vi "Update Clock Map.vi"(7 "Reset":bool, 9 "ClockID":u8, 10 "Timestamp Pair":T1, 11 "Clock History Map in":T3) -> (3 "Clock History Map out":map{u8, T2}(c390))   [LabVIEW 2021, in "CIFClocks.lvlib"]
uses:
  CIFClocks.lvlib
  Typedef/Clock History Map.ctl
  Typedef/Clock History.ctl
  Typedef/Timestamp Pair.ctl
  <vilib>/Utility/miscctls.llb/LVMapReplaceAction.ctl
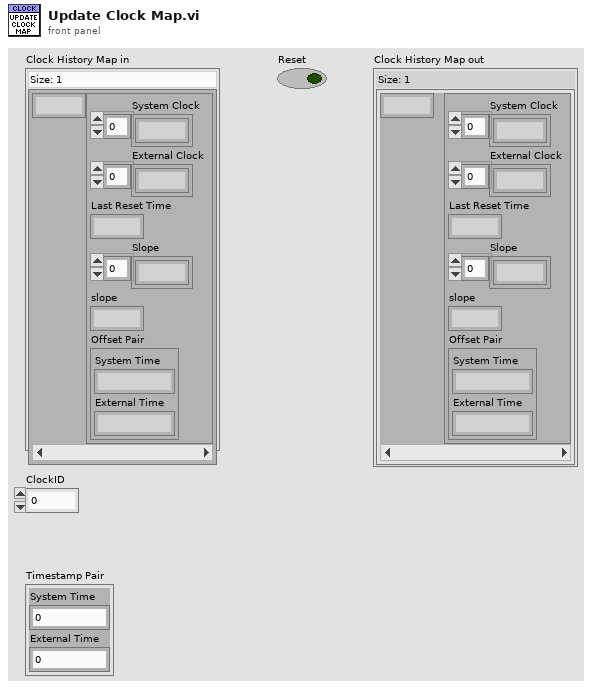
[diagram p1: front panel]
types:
  T1 = typedef "CIFClocks.lvlib/Timestamp Pair.ctl" = cluster{"System Time":i64, "External Time":i64}
  T2 = typedef "CIFClocks.lvlib/Clock History.ctl" = cluster{"System Clock":i64[], "External Clock":i64[], "Last Reset Time":u64, "Slope":dbl[], "slope":dbl, "Offset Pair":T1}
  T3 = typedef "CIFClocks.lvlib/Clock History Map.ctl" = map{u8, T2}
  T4 = typedef "LVMapReplaceAction.ctl" = enum32{"Modify Entry only if found", "Add or Modify Entry", "Delete Entry"}
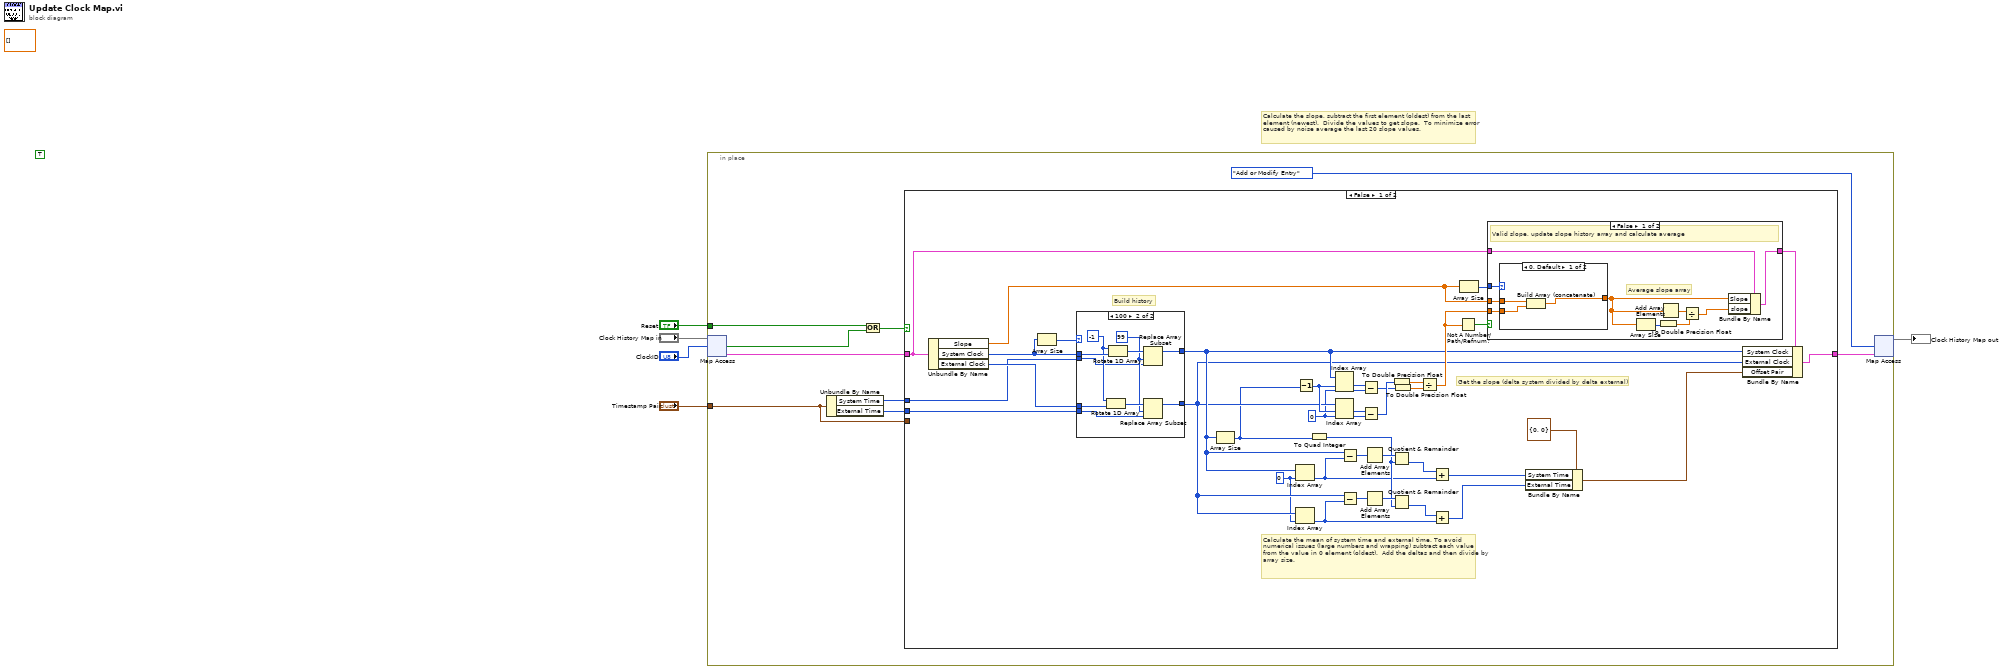
[diagram p0: block diagram]
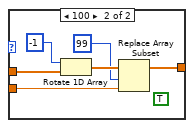
[diagram p2: hidden frame]
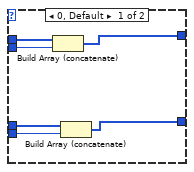
[diagram p4: hidden frame]
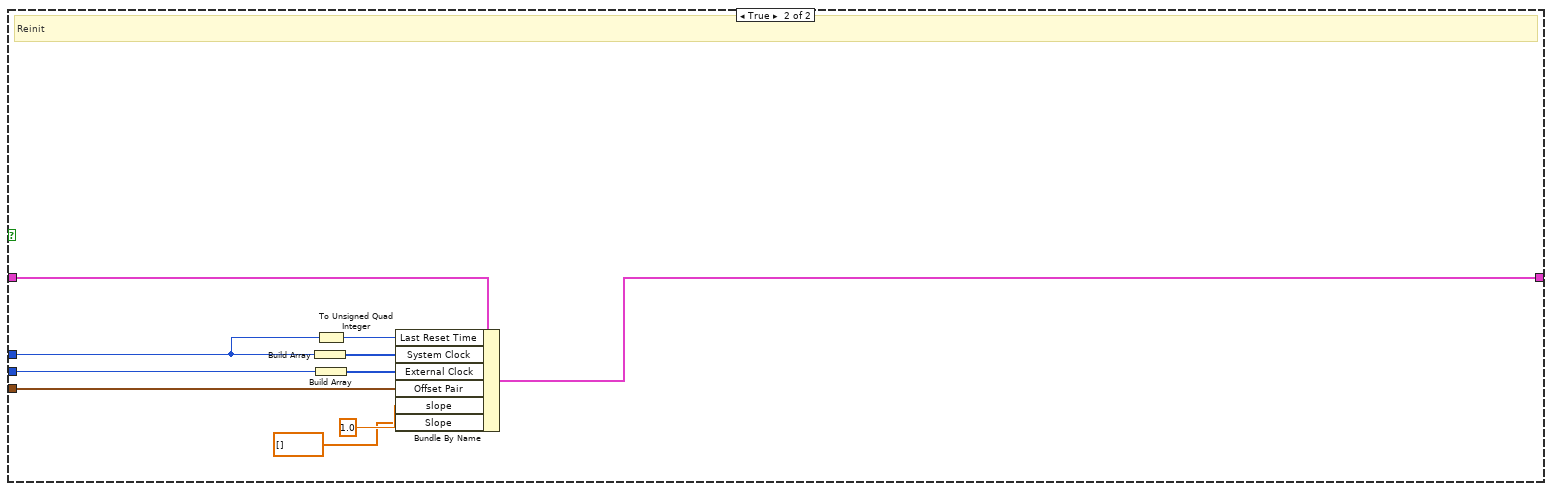
[diagram p5: hidden frame]
diagram:
  (unwired) TRUE
  (unwired) dbl[][] []
  # "Calculate the slope, subtract the first element (oldest) from the last element (newest).  Divide the values to get slope.  To minimize error caused by noise average the last 20 slope values."
  n1 = in-place {
    in-place-border: "Timestamp Pair" -> [w6]
    in-place-border: "Reset" -> [w13]
    n2 = in-place-map #1("Clock History Map in", "ClockID") -> (w11:T2, w14:bool)  [unwired: 1 in]
    n3 = Unbundle By Name(w6) -> ("System Time"=w8:i64, "External Time"=w7:i64)
    n4 = Or(x=w13, y=w14) -> (x .or. y?=w12:bool)
    n5 = case shown="False" w12 {
      tunnel: w11 -> [w31 w99]
      tunnel: [w29 w96] -> w10
      tunnel: w8 -> [w50 w94]
      tunnel: w7 -> [w49 w95]
      tunnel: w6 -> [_ w92]
      frame False {
        w19 = 0 ("index")
        w15 = 0 ("index")
        # "Calculate the mean of system time and external time. To avoid numerical issues (large numbers and wrapping) subtract each value from the value in 0 element (oldest).  Add the deltas and then divide by array size."
        # "Get the slope (delta system divided by delta external)"
        # "Build history"
        n6 = Unbundle By Name(w31) -> ("Slope"=w36:dbl[], "System Clock"=w51:i64[], "External Clock"=w52:i64[])
        n7 = Array Size(array=w51) -> (size(s)=w53:i32)
        n8 = case shown="100" w53 {
          tunnel: w52 -> [w77 w89]
          tunnel: w51 -> [w79 w88]
          tunnel: [w78 w83] -> w28
          tunnel: [w76 w82] -> w27
          tunnel: w50 -> [w75 w80]
          tunnel: w49 -> [w74 w81]
          frame 0, Default {
            n9 = Build Array (concatenate)(w79, w75) -> (w78:i64[])
            n10 = Build Array (concatenate)(w77, w74) -> (w76:i64[])
          }
          frame 100 {
            w84 = 99 ("index")
            w87 = -1 ("n")
            n11 = Rotate 1D Array(1:w89, 2:w87) -> (0:w86:i64[])
            n12 = Rotate 1D Array(1:w88, 2:w87) -> (0:w85:i64[])
            n13 = Replace Array Subset(array=w85, new element=w80, index=w84) -> (w83:i64[])
            n14 = Replace Array Subset(array=w86, new element=w81, index=w84) -> (w82:i64[])
          }
        }
        n15 = Array Size(array=w28) -> (size(s)=w16:i32)
        n16 = Index Array(array=w28, index=w19) -> (element=w17:i64)
        n17 = Index Array(array=w27, index=w19) -> (element=w18:i64)
        n18 = Decrement(x=w16) -> (x-1=w33:i32)
        n19 = To Quad Integer(1:w16) -> (0:w20:i64)
        n20 = Index Array(array=w28, index #1=w33, index #2=w15) -> (element #1=w48:i64, element #2=w47:i64)
        n21 = Index Array(array=w27, index #1=w33, index #2=w15) -> (element #1=w45:i64, element #2=w46:i64)
        n22 = Subtract(x=w28, y=w17) -> (x-y=w26:i64[])
        n23 = Subtract(x=w27, y=w18) -> (x-y=w21:i64[])
        n24 = Subtract(x=w48, y=w47) -> (x-y=w43:i64)
        n25 = Subtract(x=w45, y=w46) -> (x-y=w44:i64)
        n26 = Add Array Elements(numeric array=w26) -> (sum=w25:i64)
        n27 = Add Array Elements(numeric array=w21) -> (sum=w22:i64)
        n28 = To Double Precision Float(number=w44) -> (double precision float=w40:dbl)
        n29 = Quotient & Remainder(x=w25, y=w20) -> (floor(x/y)=w24:i64)  [unwired: 1 out]
        n30 = Quotient & Remainder(x=w22, y=w20) -> (floor(x/y)=w23:i64)  [unwired: 1 out]
        n31 = To Double Precision Float(number=w43) -> (double precision float=w39:dbl)
        n32 = Divide(x=w40, y=w39) -> (x/y=w32:dbl)
        n33 = Add(x=w24, y=w17) -> (x+y=w38:i64)
        n34 = Add(x=w23, y=w18) -> (x+y=w37:i64)
        n35 = Not A Number/Path/Refnum?(number/path/refnum=w32) -> (NaN/Path/Refnum?=w34:bool)
        n36 = Array Size(array=w36) -> (size(s)=w35:i32)
        n37 = case shown="False" w34 {
          tunnel: w36 -> [w63 _]
          tunnel: w32 -> [w62 _]
          tunnel: w35 -> [w61 _]
          tunnel: w31 -> [w57 w73]
          tunnel: [w54 w73] -> w30
          frame False {
            # "Average slope array"
            # "Valid slope, update slope history array and calculate average"
            n38 = case shown="0, Default" w61 {
              tunnel: w63 -> [w66 w72]
              tunnel: [w65 w68] -> w55
              tunnel: w62 -> [w64 w67]
              frame 0, Default {
                n39 = Build Array (concatenate)(w66, w64) -> (w65:dbl[])
              }
              frame 100 {
                (unwired) TRUE
                n40 = Rotate 1D Array(1:w72, 2:-1 ("n")) -> (0:w70:dbl[])
                n41 = Replace Array Subset(array=w70, new element=w67, index=99) -> (w68:dbl[])
              }
            }
            n42 = Array Size(array=w55) -> (size(s)=w60:i32)
            n43 = To Double Precision Float(number=w60) -> (double precision float=w58:dbl)
            n44 = Add Array Elements(numeric array=w55) -> (sum=w59:dbl)
            n45 = Divide(x=w59, y=w58) -> (x/y=w56:dbl)
            n46 = Bundle By Name(cluster=w57, "Slope"=w55, "slope"=w56) -> (w54:T2)
          }
          frame True {
            # "NaN, don't change slope"
          }
        }
        n47 = Bundle By Name(cluster=T1 {"System Time"=0, "External Time"=0} ("Offset Pair"), "System Time"=w38, "External Time"=w37) -> (w41:T1)
        n48 = Bundle By Name(cluster=w30, "System Clock"=w28, "External Clock"=w27, "Offset Pair"=w41) -> (w29:T2)
      }
      frame True {
        # "Reinit"
        n49 = Build Array(w94) -> (w98:i64[])
        n50 = To Unsigned Quad Integer(1:w94) -> (0:w91:u64)
        n51 = Build Array(w95) -> (w97:i64[])
        n52 = Bundle By Name(cluster=w99, "Last Reset Time"=w91, "System Clock"=w98, "External Clock"=w97, "Offset Pair"=w92, "slope"=1.0, "Slope"=dbl[] []) -> (w96:T2)
      }
    }
    n53 = in-place-map #1(w10, LVMapReplaceAction."Add or Modify Entry" ("action")) -> (→"Clock History Map out":T3)  [unwired: 2 out]
  }
